vi "Demo.vi"() -> ()   [LabVIEW 2009]
uses:
  MVCAMSDK.dll
panel:
  in  "Stop 2":bool
  out "Video 2":T1(plugin-control)
  in  "显示相机参数面板 2":bool
  in  "拍照 2":bool
  in  "激活预览 2":bool
  in  "要写入相机2的字符串(32字节)":string
  in  "写入自定义数据 2":bool
  out "从相机2中读出的字符串(32字节)":string
  in  "读取自定义数据 2":bool
  out "Video":T1(plugin-control)
  in  "读取自定义数据":bool
  out "从相机1中读出的字符串(32字节)":string
  in  "写入自定义数据":bool
  in  "要写入相机1的字符串(32字节)":string
  in  "拍照":bool
  in  "显示相机参数面板":bool
  in  "Stop":bool
  in  "激活预览":bool
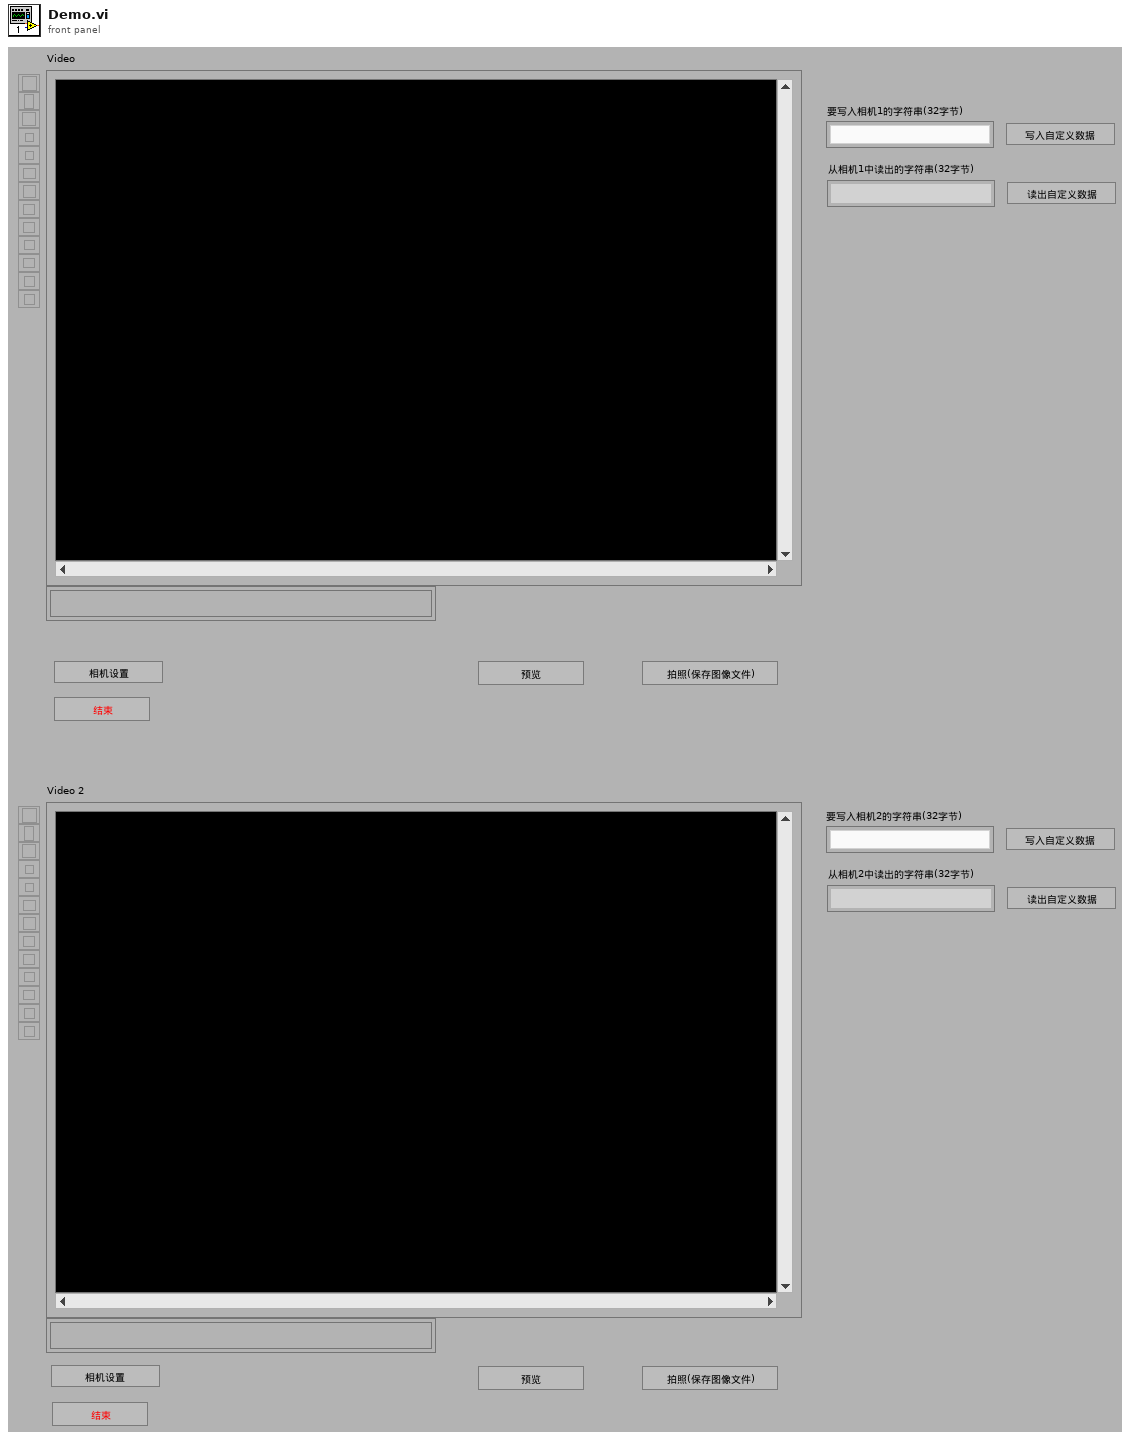
[diagram p1: front panel]
types:
  T1 = typedef "IMAQ Image.ctl" = refnum<image>
  T2 = typedef "Image Type" = u32
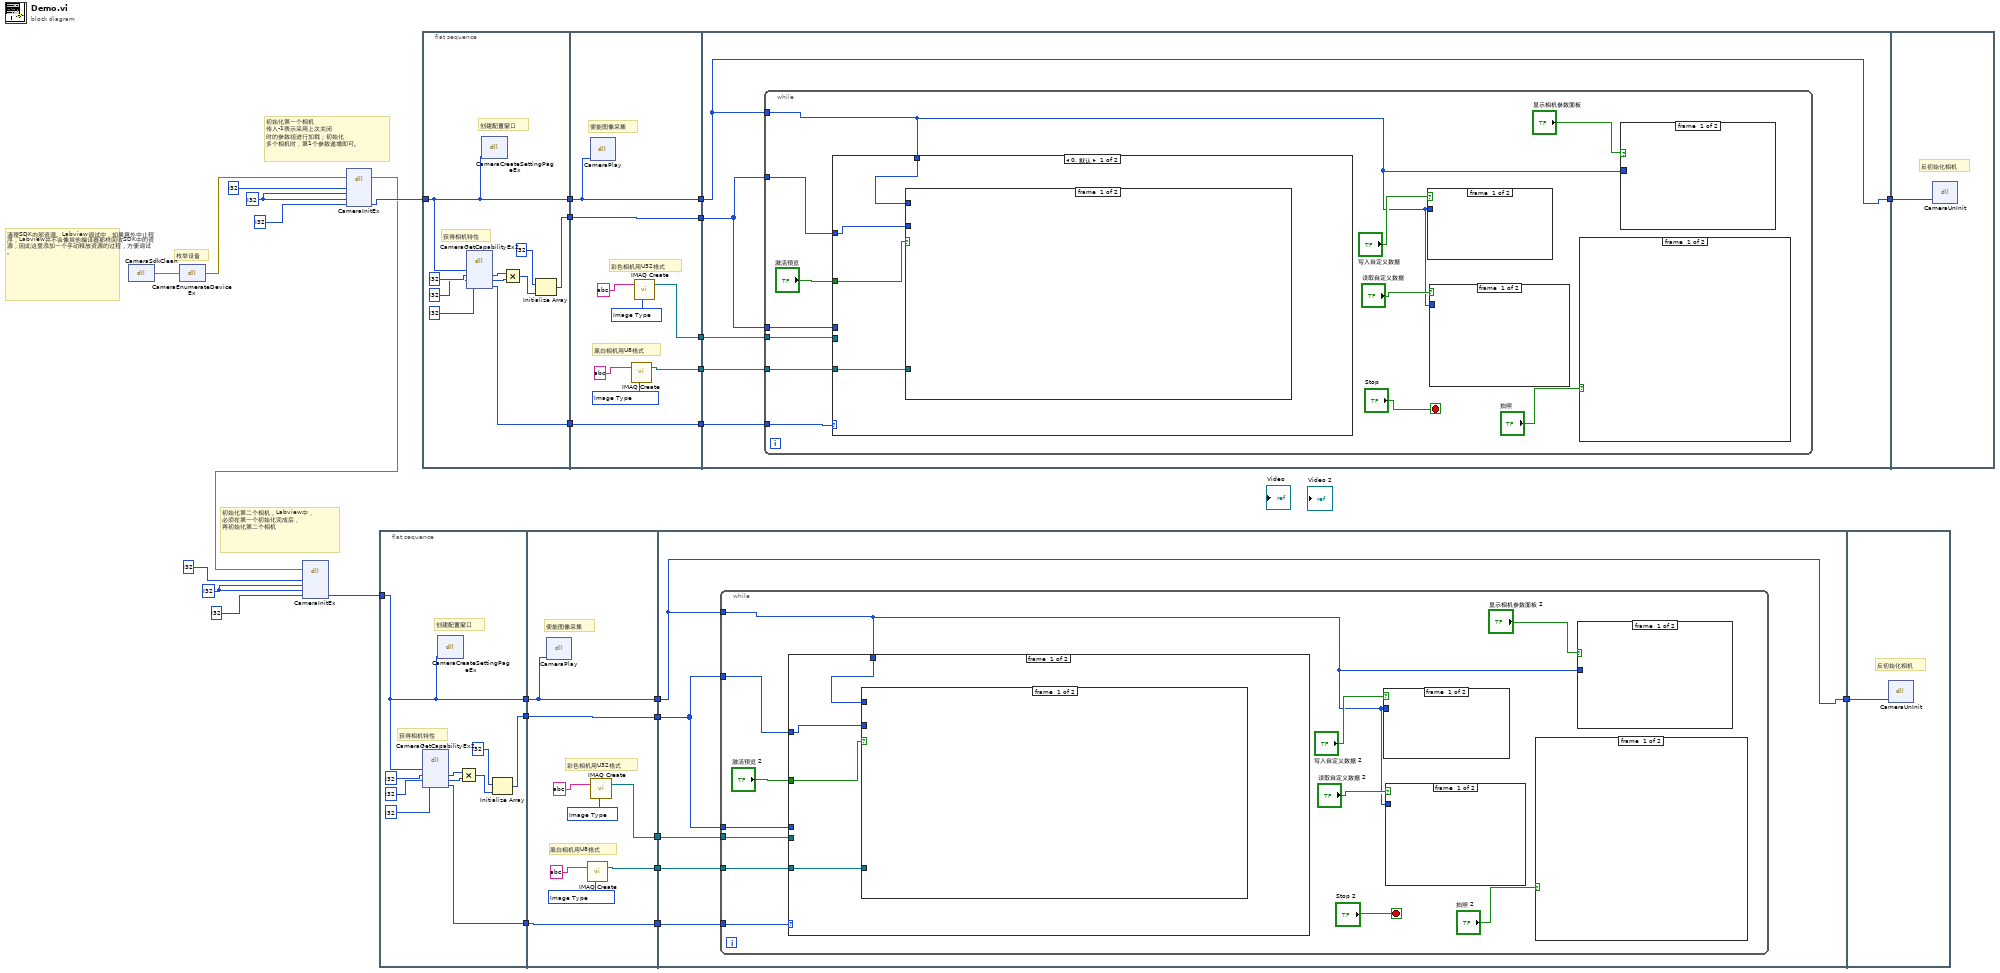
[diagram p0: block diagram]
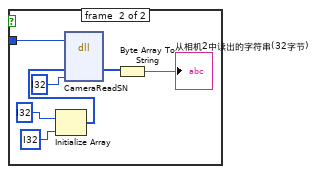
[diagram p2: hidden frame]
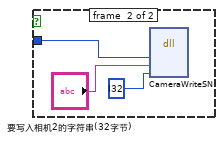
[diagram p3: hidden frame]
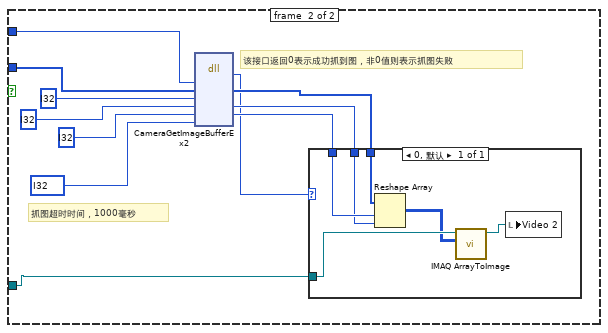
[diagram p4: hidden frame]
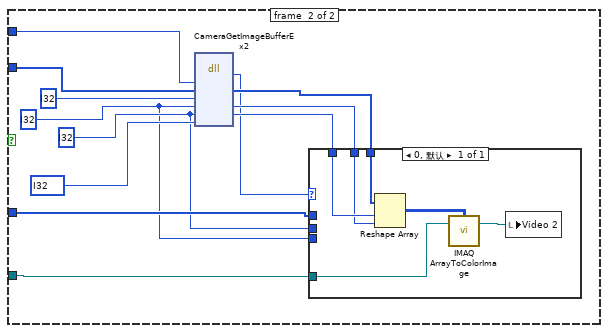
[diagram p6: hidden frame]
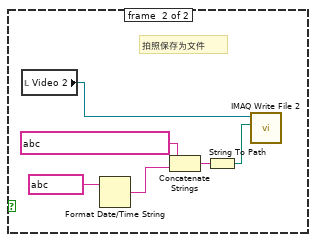
[diagram p7: hidden frame]
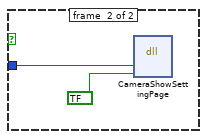
[diagram p8: hidden frame]
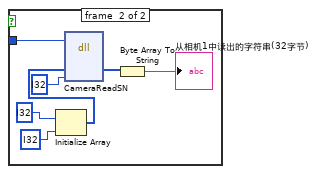
[diagram p9: hidden frame]
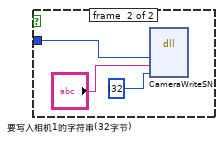
[diagram p10: hidden frame]
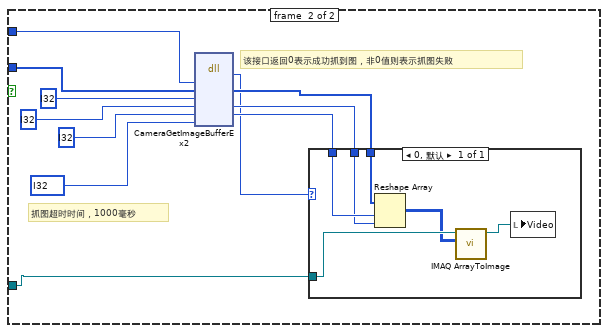
[diagram p11: hidden frame]
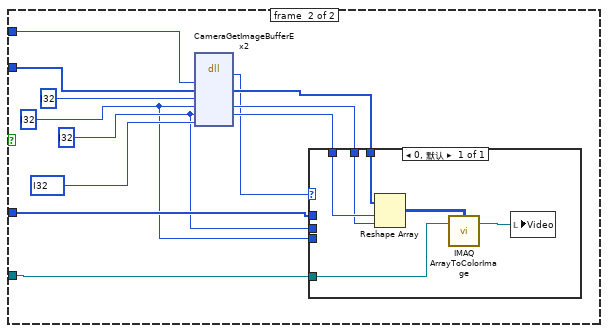
[diagram p13: hidden frame]
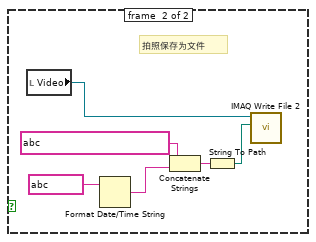
[diagram p14: hidden frame]
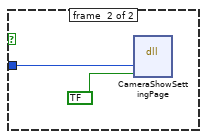
[diagram p15: hidden frame]
diagram:
  w5 = i32 ?
  w10 = i32 ?
  # "枚举设备"
  # "初始化第一个相机\n传入-1表示采用上次关闭\n时的参数组进行加载；初始化\n多个相机时，第1个参数递增即可。"
  # "初始化第二个相机，Labview中，\n必须在第一个初始化完成后，\n再初始化第二个相机"
  # "清理SDK内部资源。Labview调试中，如果意外中止程序，Labview并不会像其他编译器那样回收SDK中的资源，因此这里添加一个手动释放资源的过程，方便调试。"
  n1 = dll-call lib="MVCAMSDK.dll" fn="CameraSdkClean"() -> (error out=w11:errorcluster)  [unwired: 4 in, 1 out]
  n2 = dll-call lib="MVCAMSDK.dll" fn="CameraEnumerateDeviceEx"(error in=w11) -> (error out=w2:errorcluster)  [unwired: 3 in, 1 out]
  n3 = dll-call lib="MVCAMSDK.dll" fn="CameraInitEx"(error in=w2, "相机索引值"=i32 ?, "参数加载方式"=w5, "要加载的参数组索引"=w5, "相机句柄"=i32 ?) -> (error out=w1:errorcluster, "相机句柄"=w3:i32)  [unwired: 6 in, 1 out]
  n4 = dll-call lib="MVCAMSDK.dll" fn="CameraInitEx"(error in=w1, "相机索引值"=i32 ?, "参数加载方式"=w10, "要加载的参数组索引"=w10, "相机句柄"=i32 ?) -> ("相机句柄"=w4:i32)  [unwired: 6 in, 2 out]
  n5 = flat-sequence {
    tunnel: [w30] -> w20
    tunnel: [w37] -> w19
    tunnel: [w31] -> w18
    tunnel: w4 -> [w30]
    tunnel: w20 -> [w48]
    tunnel: [w48] -> w17
    tunnel: [w45] -> w16
    tunnel: w19 -> [w44]
    tunnel: [w44] -> w15
    tunnel: w18 -> [w43]
    tunnel: [w43] -> w14
    tunnel: [w40] -> w13
    tunnel: w17 -> [w51]
    tunnel: [w51] -> w12
    tunnel: w16 -> [w53]
    tunnel: w15 -> [w49]
    tunnel: w14 -> [w52]
    tunnel: w13 -> [w50]
    tunnel: w12 -> [w128]
    frame #0 {
      # "获得相机特性"
      # "创建配置窗口"
      n6 = dll-call lib="MVCAMSDK.dll" fn="CameraGetCapabilityEx2"("相机句柄"=w30, "图像最大宽度"=i32 ?, "图像最大高度"=i32 ?, "是否是彩色相机(返回0:黑白;1:彩色)"=i32 ?) -> ("图像最大宽度"=w33:i32, "图像最大高度"=w32:i32, "是否是彩色相机(返回0:黑白;1:彩色)"=w31:i32)  [unwired: 5 in, 2 out]
      n7 = dll-call lib="MVCAMSDK.dll" fn="CameraCreateSettingPageEx"("相机句柄"=w30) -> ()  [unwired: 5 in, 2 out]
      n8 = Multiply(x=w33, y=w32) -> (x*y=w38:i32)
      n9 = Initialize Array(i32 ?, w38) -> (w37:i32[])
    }
    frame #1 {
      w42 = T2 ? items=["Grayscale (U8)", "Grayscale (I16)", "Grayscale (SGL)", "Complex (CSG)", "RGB (U32)", "HSL (U32)", "RGB (U64)", "Grayscale (U16)"] ("Image Type")
      w47 = T2 ? items=["Grayscale (U8)", "Grayscale (I16)", "Grayscale (SGL)", "Complex (CSG)", "RGB (U32)", "HSL (U32)", "RGB (U64)", "Grayscale (U16)"] ("Image Type")
      # "黑白相机用U8格式"
      # "彩色相机用U32格式"
      # "使能图像采集"
      n10 = dll-call lib="MVCAMSDK.dll" fn="CameraPlay"("相机句柄"=w48) -> ()  [unwired: 5 in, 2 out]
      n11 = call "IMAQ Create"("Image Name"=string ?, "Image Type"=w42) -> ("New Image"=w40:T1)  [unwired: 3 in, 1 out]
      n12 = call "IMAQ Create"("Image Name"=string ?, "Image Type"=w47) -> ("New Image"=w45:T1)  [unwired: 3 in, 1 out]
    }
    frame #2 {
      n13 = while {
        tunnel: w51 -> [w55]
        tunnel: w53 -> [w62]
        tunnel: w49 -> [w63]
        tunnel: w52 -> [w61]
        tunnel: w50 -> [w59]
        tunnel: w49 -> [w58]
        stop <- "Stop 2" stop-if-true
        n14 = case shown="1" w61 {
          tunnel: w63 -> [w77 w101]
          tunnel: w62 -> [_ w98]
          tunnel: w55 -> [w78 w100]
          tunnel: "激活预览 2" -> [w76 w99]
          tunnel: w59 -> [w79 _]
          tunnel: w58 -> [_ w97]
          frame #0 {
            n15 = case shown="真" w76 {
              tunnel: w78 -> [_ w90]
              tunnel: w77 -> [_ w81]
              tunnel: w79 -> [_ w80]
              frame #0 {
              }
              frame #1 {
                # "该接口返回0表示成功抓到图，非0值则表示抓图失败"
                # "抓图超时时间，1000毫秒"
                n16 = dll-call lib="MVCAMSDK.dll" fn="CameraGetImageBufferEx2"("相机句柄"=w90, "图像数据缓冲区"=w81, "图像输出格式(0:8位灰度;1:24位彩色;2:32位彩色)"=i32 ?, "图像宽度"=i32 ?, "图像高度"=i32 ?, "抓图超时时间(毫秒)"=i32 ?) -> ("返回类型"=w82:i32, "图像数据缓冲区"=w85:u8[], "图像宽度"=w83:i32, "图像高度"=w84:i32)  [unwired: 6 in, 2 out]
                n17 = case shown="0, 默认" w82 {
                  tunnel: w85 -> [w96]
                  tunnel: w80 -> [w93]
                  tunnel: w84 -> [w95]
                  tunnel: w83 -> [w94]
                  frame 0, 默认 {
                    n18 = Reshape Array(w96, w95, w94) -> (w92:u8[][])
                    n19 = call "IMAQ ArrayToImage"("Image Pixels (U8)"=w92, "Image"=w93) -> ("Image Out"=w91:T1)  [unwired: 8 in, 1 out]
                    n20 = local write "Video 2"(w91) -> ()
                  }
                }
              }
            }
          }
          frame #1 {
            n21 = case shown="真" w99 {
              tunnel: w100 -> [_ w113]
              tunnel: w98 -> [_ w106]
              tunnel: w101 -> [_ w105]
              tunnel: w97 -> [_ w104]
              frame #0 {
              }
              frame #1 {
                w102 = i32 ?
                w103 = i32 ?
                n22 = dll-call lib="MVCAMSDK.dll" fn="CameraGetImageBufferEx2"("相机句柄"=w113, "图像数据缓冲区"=w105, "图像输出格式(0:8位灰度;1:24位彩色;2:32位彩色)"=i32 ?, "图像宽度"=w102, "图像高度"=w103, "抓图超时时间(毫秒)"=i32 ?) -> ("返回类型"=w107:i32, "图像数据缓冲区"=w110:u32[], "图像宽度"=w108:i32, "图像高度"=w109:i32)  [unwired: 6 in, 2 out]
                n23 = case shown="0, 默认" w107 {
                  tunnel: w110 -> [w117]
                  tunnel: w106 -> [w116]
                  tunnel: w109 -> [w115]
                  tunnel: w108 -> [w114]
                  tunnel: w104 -> [_]
                  tunnel: w103 -> [_]
                  tunnel: w102 -> [_]
                  frame 0, 默认 {
                    n24 = Reshape Array(w117, w115, w114) -> (w118:u32[][])
                    n25 = call "IMAQ ArrayToColorImage"("Image Pixels (U32)"=w118, "Image"=w116) -> ("Image Out"=w119:T1)  [unwired: 3 in, 1 out]
                    n26 = local write "Video 2"(w119) -> ()
                  }
                }
              }
            }
          }
        }
        n27 = case shown="真" "写入自定义数据 2" {
          tunnel: w55 -> [_ w75]
          frame #0 {
          }
          frame #1 {
            n28 = dll-call lib="MVCAMSDK.dll" fn="CameraWriteSN"("相机句柄"=w75, "序列号(固定为32个字节)"="要写入相机2的字符串(32字节)", "序列号级别，[0,1,2]对应3级序列号，其中0级为只读，1,2级可写"=i32 ?) -> ()  [unwired: 7 in, 2 out]
          }
        }
        n29 = case shown="真" "读取自定义数据 2" {
          tunnel: w55 -> [_ w72]
          frame #0 {
          }
          frame #1 {
            n30 = Initialize Array(i32 ?, i32 ?) -> (w69:i32[])
            n31 = dll-call lib="MVCAMSDK.dll" fn="CameraReadSN"("相机句柄"=w72, "序列号"=w69, "序列号级别，[0,1,2],0级为只读，1,2级可写"=i32 ?) -> ("序列号"=w67:u8[])  [unwired: 6 in, 2 out]
            n32 = Byte Array To String(unsigned byte array=w67) -> (string=→"从相机2中读出的字符串(32字节)":string)
          }
        }
        n33 = case shown="真" "拍照 2" {
          frame #0 {
          }
          frame #1 {
            # "拍照保存为文件"
            n34 = local read "Video 2"() -> (w120:T1)
            n35 = Format Date/Time String(time format string (%c)=string ?) -> (date/time string=w124:string)  [unwired: 2 in]
            n36 = Concatenate Strings(string ?, w124) -> (w121:string)
            n37 = String To Path(string=w121) -> (path=w123:path)
            n38 = call-poly "IMAQ Write File 2"("File Path"=w123, "Image"=w120) -> ()  [unwired: 8 in, 2 out]
          }
        }
        n39 = case shown="真" "显示相机参数面板 2" {
          tunnel: w55 -> [_ w127]
          frame #0 {
          }
          frame #1 {
            n40 = dll-call lib="MVCAMSDK.dll" fn="CameraShowSettingPage"("相机句柄"=w127, "状态"=bool ?) -> ()  [unwired: 6 in, 2 out]
          }
        }
      }
    }
    frame #3 {
      # "反初始化相机"
      n41 = dll-call lib="MVCAMSDK.dll" fn="CameraUnInit"("相机句柄"=w128) -> ()  [unwired: 5 in, 2 out]
    }
  }
  n42 = flat-sequence {
    tunnel: [w129] -> w26
    tunnel: [w136] -> w25
    tunnel: [w130] -> w23
    tunnel: w3 -> [w129]
    tunnel: w26 -> [w147]
    tunnel: [w147] -> w29
    tunnel: [w144] -> w27
    tunnel: w25 -> [w143]
    tunnel: [w143] -> w24
    tunnel: w23 -> [w142]
    tunnel: [w142] -> w22
    tunnel: [w139] -> w21
    tunnel: w29 -> [w150]
    tunnel: [w150] -> w28
    tunnel: w27 -> [w152]
    tunnel: w24 -> [w148]
    tunnel: w22 -> [w151]
    tunnel: w21 -> [w149]
    tunnel: w28 -> [w227]
    frame #0 {
      # "获得相机特性"
      # "创建配置窗口"
      n43 = dll-call lib="MVCAMSDK.dll" fn="CameraGetCapabilityEx2"("相机句柄"=w129, "图像最大宽度"=i32 ?, "图像最大高度"=i32 ?, "是否是彩色相机(返回0:黑白;1:彩色)"=i32 ?) -> ("图像最大宽度"=w132:i32, "图像最大高度"=w131:i32, "是否是彩色相机(返回0:黑白;1:彩色)"=w130:i32)  [unwired: 5 in, 2 out]
      n44 = dll-call lib="MVCAMSDK.dll" fn="CameraCreateSettingPageEx"("相机句柄"=w129) -> ()  [unwired: 5 in, 2 out]
      n45 = Multiply(x=w132, y=w131) -> (x*y=w137:i32)
      n46 = Initialize Array(i32 ?, w137) -> (w136:i32[])
    }
    frame #1 {
      w141 = T2 ? items=["Grayscale (U8)", "Grayscale (I16)", "Grayscale (SGL)", "Complex (CSG)", "RGB (U32)", "HSL (U32)", "RGB (U64)", "Grayscale (U16)"] ("Image Type")
      w146 = T2 ? items=["Grayscale (U8)", "Grayscale (I16)", "Grayscale (SGL)", "Complex (CSG)", "RGB (U32)", "HSL (U32)", "RGB (U64)", "Grayscale (U16)"] ("Image Type")
      # "黑白相机用U8格式"
      # "彩色相机用U32格式"
      # "使能图像采集"
      n47 = dll-call lib="MVCAMSDK.dll" fn="CameraPlay"("相机句柄"=w147) -> ()  [unwired: 5 in, 2 out]
      n48 = call "IMAQ Create"("Image Name"=string ?, "Image Type"=w141) -> ("New Image"=w139:T1)  [unwired: 3 in, 1 out]
      n49 = call "IMAQ Create"("Image Name"=string ?, "Image Type"=w146) -> ("New Image"=w144:T1)  [unwired: 3 in, 1 out]
    }
    frame #2 {
      n50 = while {
        tunnel: w150 -> [w154]
        tunnel: w152 -> [w161]
        tunnel: w148 -> [w162]
        tunnel: w151 -> [w160]
        tunnel: w149 -> [w158]
        tunnel: w148 -> [w157]
        stop <- "Stop" stop-if-true
        n51 = case shown="0, 默认" w160 {
          tunnel: w162 -> [w176 w200]
          tunnel: w161 -> [_ w197]
          tunnel: w154 -> [w177 w199]
          tunnel: "激活预览" -> [w175 w198]
          tunnel: w158 -> [w178 _]
          tunnel: w157 -> [_ w196]
          frame #0 {
            n52 = case shown="真" w175 {
              tunnel: w177 -> [_ w189]
              tunnel: w176 -> [_ w180]
              tunnel: w178 -> [_ w179]
              frame #0 {
              }
              frame #1 {
                # "该接口返回0表示成功抓到图，非0值则表示抓图失败"
                # "抓图超时时间，1000毫秒"
                n53 = dll-call lib="MVCAMSDK.dll" fn="CameraGetImageBufferEx2"("相机句柄"=w189, "图像数据缓冲区"=w180, "图像输出格式(0:8位灰度;1:24位彩色;2:32位彩色)"=i32 ?, "图像宽度"=i32 ?, "图像高度"=i32 ?, "抓图超时时间(毫秒)"=i32 ?) -> ("返回类型"=w181:i32, "图像数据缓冲区"=w184:u8[], "图像宽度"=w182:i32, "图像高度"=w183:i32)  [unwired: 6 in, 2 out]
                n54 = case shown="0, 默认" w181 {
                  tunnel: w184 -> [w195]
                  tunnel: w179 -> [w192]
                  tunnel: w183 -> [w194]
                  tunnel: w182 -> [w193]
                  frame 0, 默认 {
                    n55 = Reshape Array(w195, w194, w193) -> (w191:u8[][])
                    n56 = call "IMAQ ArrayToImage"("Image Pixels (U8)"=w191, "Image"=w192) -> ("Image Out"=w190:T1)  [unwired: 8 in, 1 out]
                    n57 = local write "Video"(w190) -> ()
                  }
                }
              }
            }
          }
          frame #1 {
            n58 = case shown="真" w198 {
              tunnel: w199 -> [_ w212]
              tunnel: w197 -> [_ w205]
              tunnel: w200 -> [_ w204]
              tunnel: w196 -> [_ w203]
              frame #0 {
              }
              frame #1 {
                w201 = i32 ?
                w202 = i32 ?
                n59 = dll-call lib="MVCAMSDK.dll" fn="CameraGetImageBufferEx2"("相机句柄"=w212, "图像数据缓冲区"=w204, "图像输出格式(0:8位灰度;1:24位彩色;2:32位彩色)"=i32 ?, "图像宽度"=w201, "图像高度"=w202, "抓图超时时间(毫秒)"=i32 ?) -> ("返回类型"=w206:i32, "图像数据缓冲区"=w209:u32[], "图像宽度"=w207:i32, "图像高度"=w208:i32)  [unwired: 6 in, 2 out]
                n60 = case shown="0, 默认" w206 {
                  tunnel: w209 -> [w216]
                  tunnel: w205 -> [w215]
                  tunnel: w208 -> [w214]
                  tunnel: w207 -> [w213]
                  tunnel: w203 -> [_]
                  tunnel: w202 -> [_]
                  tunnel: w201 -> [_]
                  frame 0, 默认 {
                    n61 = Reshape Array(w216, w214, w213) -> (w217:u32[][])
                    n62 = call "IMAQ ArrayToColorImage"("Image Pixels (U32)"=w217, "Image"=w215) -> ("Image Out"=w218:T1)  [unwired: 3 in, 1 out]
                    n63 = local write "Video"(w218) -> ()
                  }
                }
              }
            }
          }
        }
        n64 = case shown="真" "写入自定义数据" {
          tunnel: w154 -> [_ w174]
          frame #0 {
          }
          frame #1 {
            n65 = dll-call lib="MVCAMSDK.dll" fn="CameraWriteSN"("相机句柄"=w174, "序列号(固定为32个字节)"="要写入相机1的字符串(32字节)", "序列号级别，[0,1,2]对应3级序列号，其中0级为只读，1,2级可写"=i32 ?) -> ()  [unwired: 7 in, 2 out]
          }
        }
        n66 = case shown="真" "读取自定义数据" {
          tunnel: w154 -> [_ w171]
          frame #0 {
          }
          frame #1 {
            n67 = Initialize Array(i32 ?, i32 ?) -> (w168:i32[])
            n68 = dll-call lib="MVCAMSDK.dll" fn="CameraReadSN"("相机句柄"=w171, "序列号"=w168, "序列号级别，[0,1,2],0级为只读，1,2级可写"=i32 ?) -> ("序列号"=w166:u8[])  [unwired: 6 in, 2 out]
            n69 = Byte Array To String(unsigned byte array=w166) -> (string=→"从相机1中读出的字符串(32字节)":string)
          }
        }
        n70 = case shown="真" "拍照" {
          frame #0 {
          }
          frame #1 {
            # "拍照保存为文件"
            n71 = local read "Video"() -> (w219:T1)
            n72 = Format Date/Time String(time format string (%c)=string ?) -> (date/time string=w223:string)  [unwired: 2 in]
            n73 = Concatenate Strings(string ?, w223) -> (w220:string)
            n74 = String To Path(string=w220) -> (path=w222:path)
            n75 = call-poly "IMAQ Write File 2"("File Path"=w222, "Image"=w219) -> ()  [unwired: 8 in, 2 out]
          }
        }
        n76 = case shown="真" "显示相机参数面板" {
          tunnel: w154 -> [_ w226]
          frame #0 {
          }
          frame #1 {
            n77 = dll-call lib="MVCAMSDK.dll" fn="CameraShowSettingPage"("相机句柄"=w226, "状态"=bool ?) -> ()  [unwired: 6 in, 2 out]
          }
        }
      }
    }
    frame #3 {
      # "反初始化相机"
      n78 = dll-call lib="MVCAMSDK.dll" fn="CameraUnInit"("相机句柄"=w227) -> ()  [unwired: 5 in, 2 out]
    }
  }
